vi "Initialize camera.vi"(4 "MASTER in":T1 {"Image data"."Color Palette" items=["Grayscale U8", "False Color", "Overexposed"]; "Image data"."Exposure time [us]" format="%#_10g"; "Queue"."Initial time [s]" format="%_19f"; "Queue"."Raw data [V]\n(all samples)" format="%0.2f"; "Queue"."Timestamp [s]" format="%_19f"}) -> (1 "MASTER out":T1 {"Image data"."Color Palette" items=["Grayscale U8", "False Color", "Overexposed"]; "Image data"."Exposure time [us]" format="%#_10g"; "Queue"."Initial time [s]" format="%_19f"; "Queue"."Raw data [V]\n(all samples)" format="%0.2f"; "Queue"."Timestamp [s]" format="%_19f"})   [LabVIEW 2020]
uses:
  MASTER.ctl
  Constants.ctl
  QBundle.ctl
  Queue.ctl
  Image data.ctl
  <vilib>/userdefined/High Color/IMAQdx.ctl
  <vilib>/vision/Image Controls.llb/IMAQ Image.ctl
  Image QBundle.ctl
  <vilib>/vision/driver/NI_Vision_Acquisition_Software.lvlib
  <resource>/objmgr/imaqdx.rc
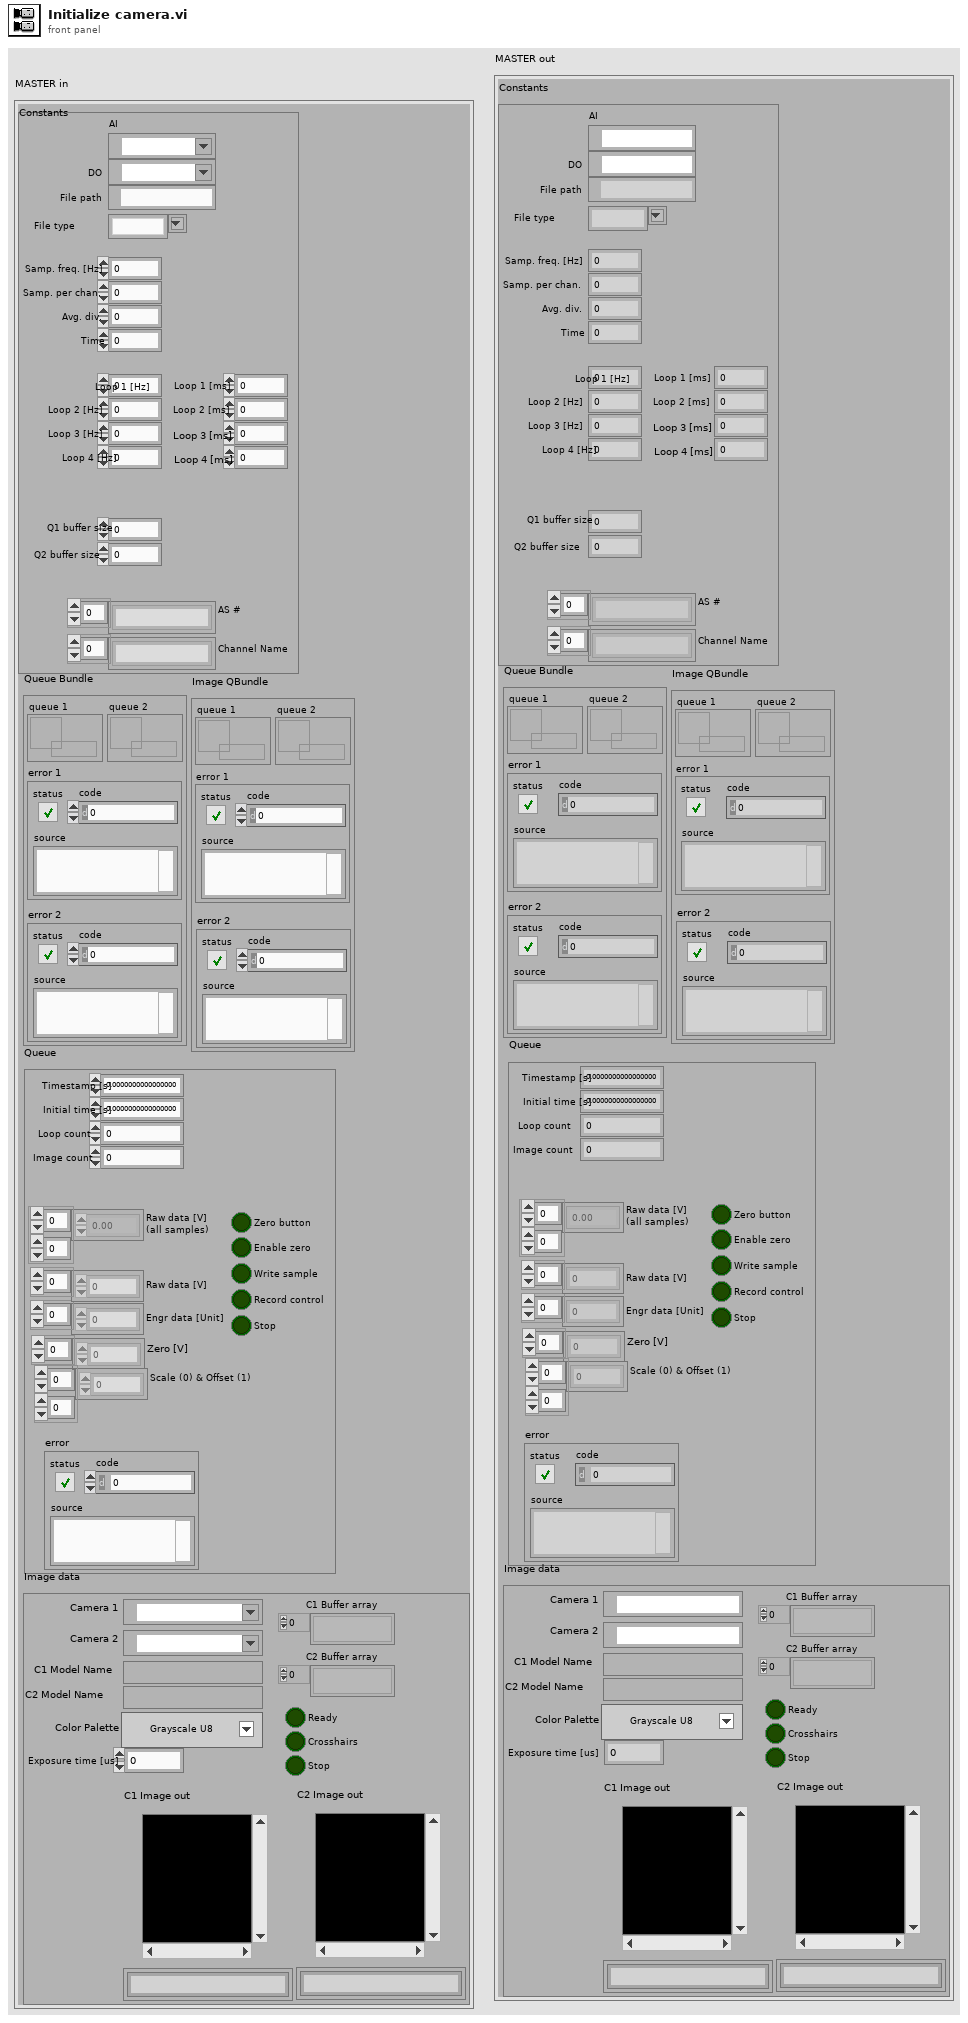
[diagram p1: front panel]
types:
  T1 = typedef "MASTER.ctl" = cluster{"Constants":T2, "Queue Bundle":T3, "Queue":T4, "Image data":T5, "Image QBundle ":T8}
  T2 = typedef "Constants.ctl" = cluster{"Time":u16, "Samp. freq. [Hz]":dbl, "Samp. per chan.":i32, "Avg. div.":i32, "File path":path, "AI":refnum<k21>, "Loop 1 [Hz]":dbl, "Loop 2 [Hz]":dbl, "Loop 3 [Hz]":dbl, "Loop 1 [ms]":dbl, "Loop 2 [ms]":dbl, "Loop 3 [ms]":dbl, "Q1 buffer size":i32, "Q2 buffer size":i32, "File type":string, "Loop 4 [Hz]":dbl, "Loop 4 [ms]":dbl, "Channel Name":string[], "AS #":string[], "DO":refnum<k21>}
  T3 = typedef "QBundle.ctl" = cluster{"queue 1":refnum<queue>, "error 1":errorcluster, "queue 2":refnum<queue>, "error 2":errorcluster}
  T4 = typedef "Queue.ctl" = cluster{"Enable zero":bool, "Engr data [Unit]":dbl[], "Zero button":bool, "Zero [V]":dbl[], "Timestamp [s]":dbl, "Write sample":bool, "Record control":bool, "Stop":bool, "error":errorcluster, "Raw data [V]\n(all samples)":dbl[][], "Raw data [V]":dbl[], "Loop count":i64, "Initial time [s]":dbl, "Scale (0) & Offset (1)":dbl[][], "Image count":dbl}
  T5 = typedef "Image data.ctl" = cluster{"Camera 1":T6, "Camera 2":T6, "C1 Image out ":T7, "C2 Image out":T7, "C1 Model Name":string, "C2 Model Name":string, "Exposure time [us]":dbl, "Color Palette":u16, "C1 Buffer array":T7[], "Ready":bool, "C2 Buffer array":T7[], "Crosshairs":bool, "Stop":bool}
  T6 = typedef "IMAQdx.ctl" = refnum<k21>
  T7 = typedef "IMAQ Image.ctl" = refnum<image>
  T8 = typedef "Image QBundle.ctl" = cluster{"queue 1":refnum<queue>, "error 1":errorcluster, "queue 2":refnum<queue>, "error 2":errorcluster}
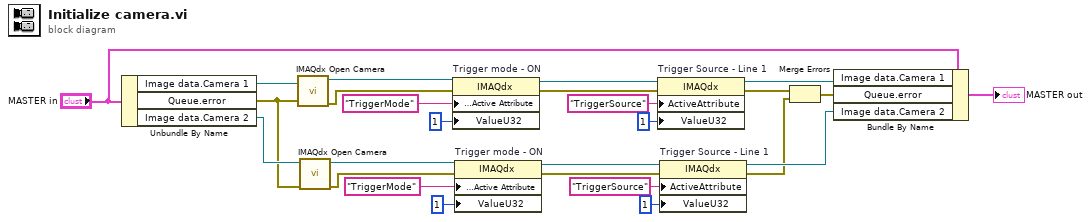
[diagram p0: block diagram]
diagram:
  n1 = Unbundle By Name("MASTER in") -> ("Image data.Camera 1"=w18:T6, "Queue.error"=w8:errorcluster, "Image data.Camera 2"=w9:T6)
  n2 = call <vilib>:"IMAQdx Open Camera.vi"("error in"=w8, "Session In"=w18) -> ("error out"=w21:errorcluster, "Session Out"=w20:T6)  [unwired: 1 in, 7 out]
  n3 = call <vilib>:"IMAQdx Open Camera.vi"("error in"=w8, "Session In"=w9) -> ("error out"=w12:errorcluster, "Session Out"=w11:T6)  [unwired: 1 in, 7 out]
  n4 = property on="Trigger mode - ON" class="IMAQdx"(reference=w20, error in=w21, "Camera Attributes:Active Attribute"="TriggerMode" ("ActiveAttribute"), "ValueU32"=u32 1) -> (reference out=w25:T6, error out=w19:errorcluster)
  n5 = property on="Trigger mode - ON" class="IMAQdx"(reference=w11, error in=w12, "Camera Attributes:Active Attribute"="TriggerMode" ("ActiveAttribute"), "ValueU32"=u32 1) -> (reference out=w16:T6, error out=w10:errorcluster)
  n6 = property on="Trigger Source - Line 1" class="IMAQdx"(reference=w25, error in=w19, "ActiveAttribute"="TriggerSource", "ValueU32"=u32 1) -> (reference out=w5:T6, error out=w2:errorcluster)
  n7 = property on="Trigger Source - Line 1" class="IMAQdx"(reference=w16, error in=w10, "ActiveAttribute"="TriggerSource", "ValueU32"=u32 1) -> (reference out=w4:T6, error out=w1:errorcluster)
  n8 = Merge Errors(w2, w1) -> (w3:errorcluster)
  n9 = Bundle By Name(cluster="MASTER in", "Image data.Camera 1"=w5, "Queue.error"=w3, "Image data.Camera 2"=w4) -> (→"MASTER out":T1)
